vi "Aux CO2 Serial Check.vi"(11 "?":T1={"Serial Port"={"termination char"=10, "End read on termination character?"=TRUE, "Enabled?"=FALSE, "VISA resource name"="COM1", "baud rate"=9600, "data bits"=8, "parity"=enum."None", "stop bits"=10, "flow control"=0, "timeout (ms)"=10000, "Input buffer size"=4096, "End write on termination character?"=TRUE, "XON Char"=17, "XOFF Char"=19}, "Baro Pressure"=760, "Device"=0} {"Device" items=["None", "TidalWave", "LoFlow / Canary", "Capnogard"]; "Serial Port"."XOFF Char" format="%.0x"; "Serial Port"."XON Char" format="%.0x"; "Serial Port"."flow control" items=["None"=0, "XON/XOFF"=1, "RTS/CTS"=2, "DTR/DSR"=4]; "Serial Port"."stop bits" items=["1.0"=10, "1.5"=15, "2.0"=20]; "Serial Port"."data bits" min=5 max=8 step=1; "Serial Port"."baud rate" items=["75"=75, "110"=110, "134"=134, "150"=150, "300"=300, "600"=600, "1200"=1200, "1800"=1800, "2400"=2400, "4800"=4800, "7200"=7200, "9600"=9600, "14400"=14400, "19200"=19200, "28800"=28800, "38400"=38400, "56000"=56000, "57600"=57600, "115200"=115200, "128000"=128000, "230400"=230400]; "Serial Port"."termination char" format="%.0x"}) -> ()   [LabVIEW 2016]
uses:
  Controls/Aux CO2 Diags.ctl
  Controls/Aux CO2 Selector.ctl
  Controls/Aux CO2 Control.ctl
  Controls/Serial Visa Control.ctl
  Controls/SerialPortControl.ctl
  Miscellaneous/Globals.vi
panel:
  in  "Set Comps":bool
  in  "Settings Cmd":bool
  in  "Zero Cmd":bool
  in  "Poff Cmd":bool
  in  "Pon Cmd":bool
  in  "Start Cmd":bool
  in  "Stop Cmd":bool
  in  "Stop Button":bool
  out "Serial Data (Hex)":string
  out "Serial Data (ASCII)":string
  out "Waveform Chart":sgl(graph)
  out "Ready to Log 2":bool
  out "Ref. Capnometer Port":T4={"Port"="", "Source"=0, "Active"=FALSE, "Baro Pressure"=760, "SerialRxBuffer"="", "Raw CO2 (Torr)"=5.0, "bytes read"=5, "Status"=[], "Status Message"=enum.""} {"Status" format="%x"; "Raw CO2 (Torr)" format="%.2f"; "Baro Pressure" min=400 max=800; "Source" items=["None", "TidalWave", "LoFlow / Canary", "Capnogard"]}
  out "Init OK":bool
  # "LoFlo Specific Commands"
  # "mmHg"
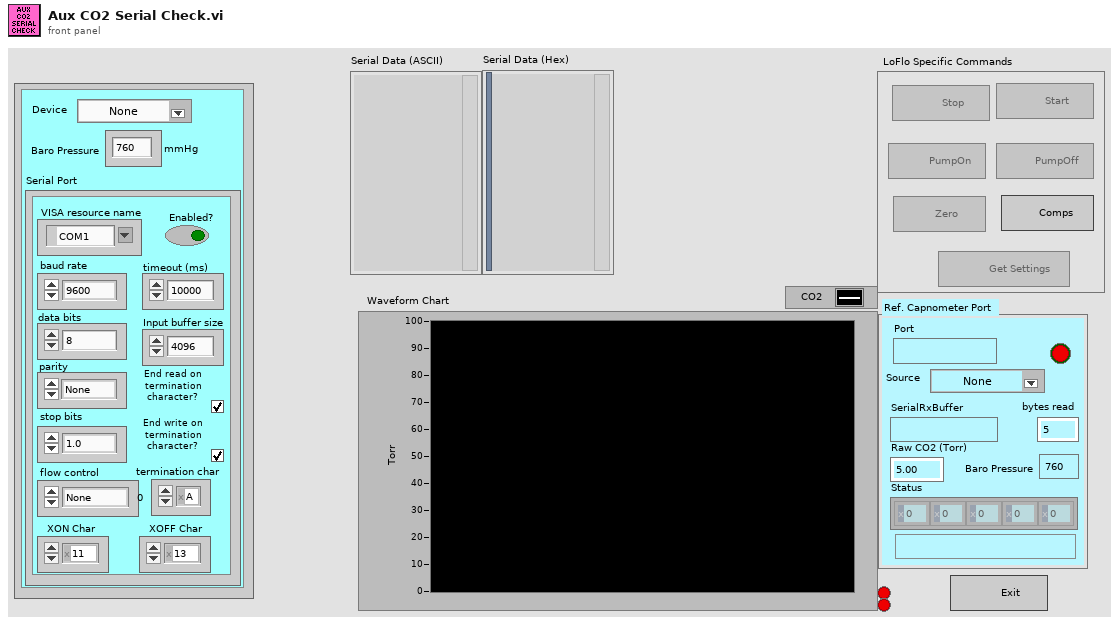
[diagram p1: front panel]
types:
  T1 = typedef "Aux CO2 Control.ctl" = cluster{"Serial Port":T2, "Baro Pressure":u32, "Device":T3}
  T2 = typedef "Serial Visa Control.ctl" = cluster{"termination char":u8, "End read on termination character?":bool, "Enabled?":bool, "VISA resource name":refnum<visa-resource-name>, "baud rate":u32, "data bits":u16, "parity":enum16{"None", "Odd", "Even", "Mark", "Space"}, "stop bits":u16, "flow control":u16, "timeout (ms)":u32, "Input buffer size":u32, "End write on termination character?":bool, "XON Char":u8, "XOFF Char":u8}
  T3 = typedef "Aux CO2 Selector.ctl" = u16
  T4 = typedef "Aux CO2 Diags.ctl" = cluster{"Port":refnum<visa-resource-name>, "Source":T3, "Active":bool, "Baro Pressure":u16, "SerialRxBuffer":string, "Raw CO2 (Torr)":sgl, "bytes read":i16, "Status":u8[], "Status Message":enum16{"", "Sensor Over Temp", "Sensor Faulty", "Set BaroP", "Capno in Sleep Mode", "Zero In Progress", "Sensor Warm Up", "Check Sampling Line", "Zero Required", "CO2 Out Of Range", "Check Airway Adapter", "LoFlo Not Connected"}}
  T5 = enum8{"Enabled", "Disabled", "Disabled and Grayed Out"}
  T6 = typedef "SerialPortControl.ctl" = enum16{"Initialize", "Write Data", "Read Data", "Close Port"}
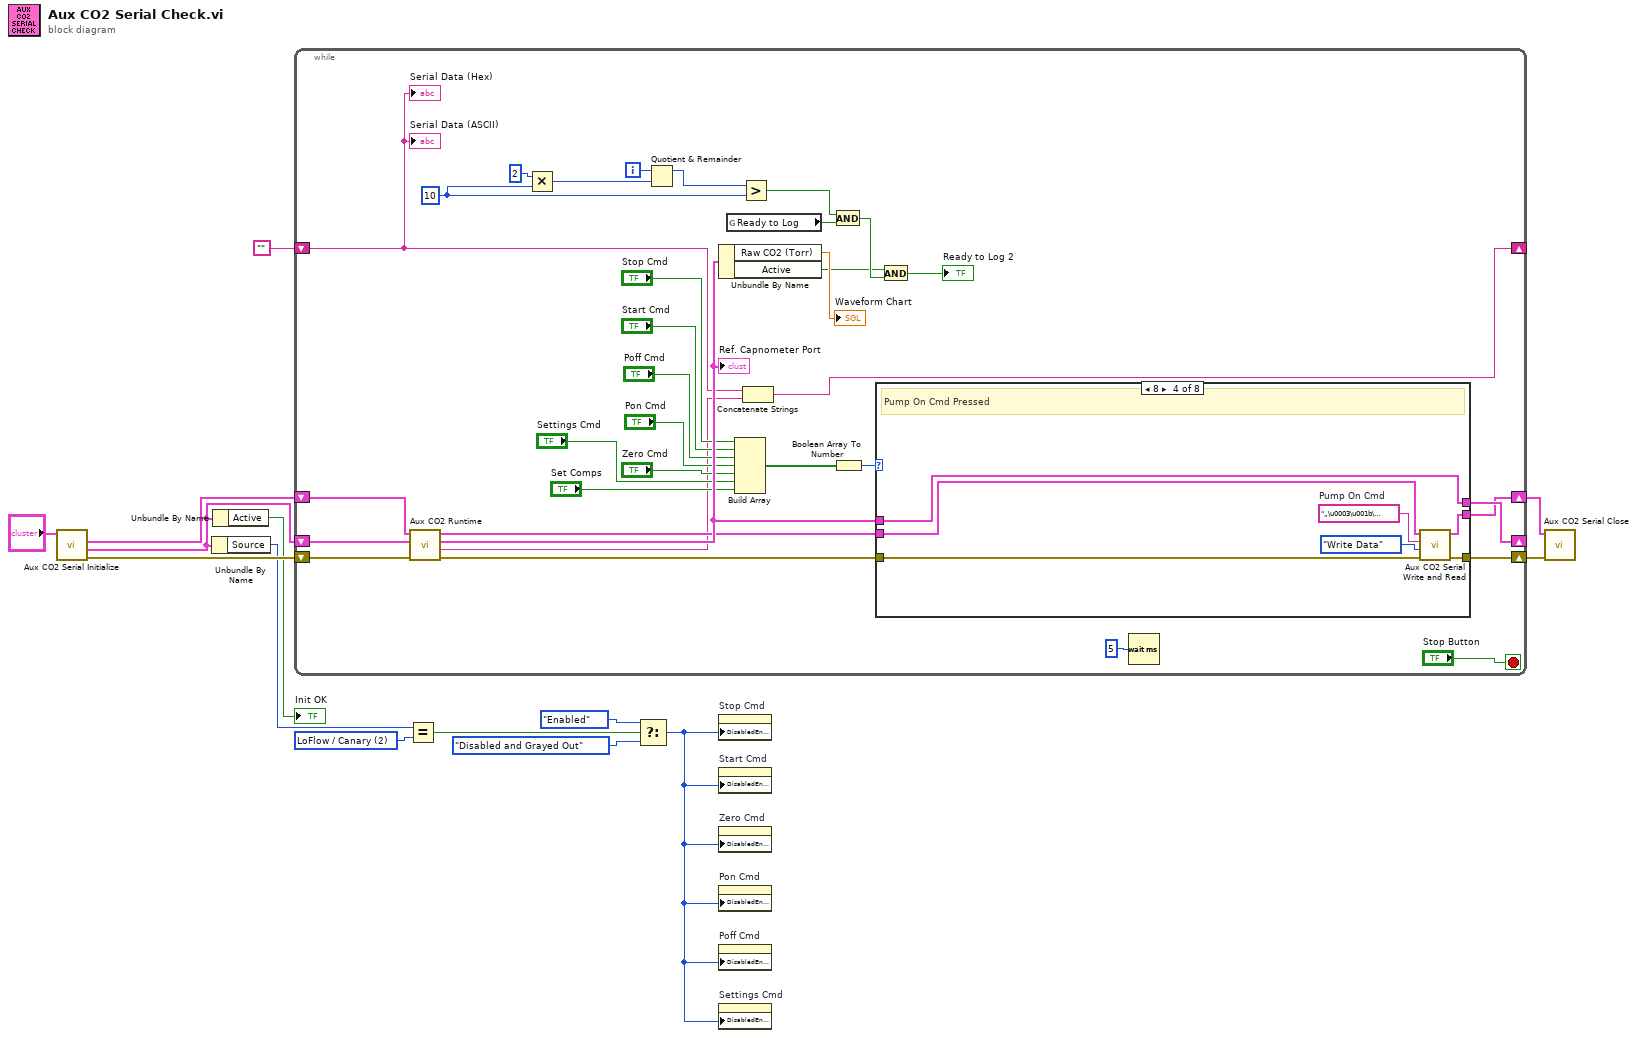
[diagram p0: block diagram]
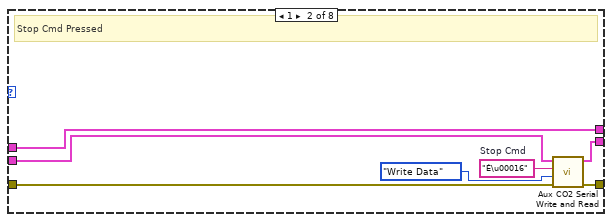
[diagram p3: hidden frame]
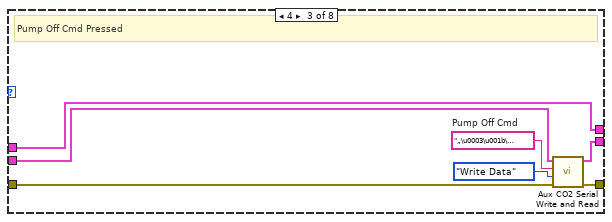
[diagram p4: hidden frame]
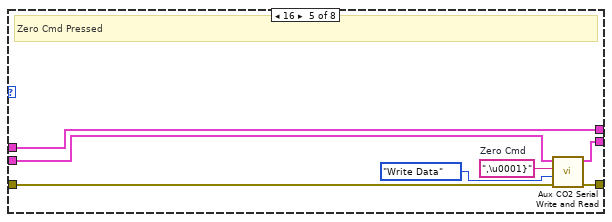
[diagram p5: hidden frame]
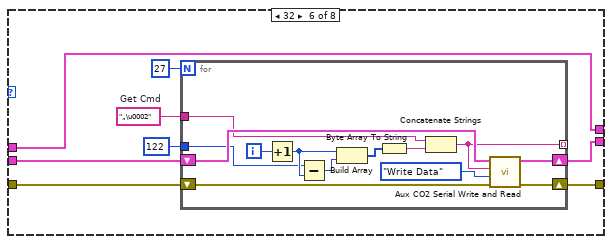
[diagram p6: hidden frame]
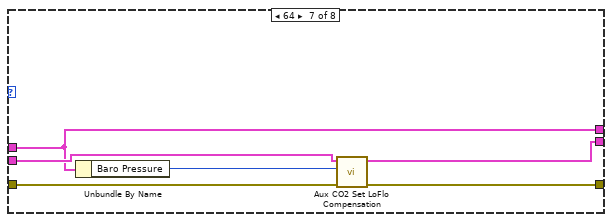
[diagram p7: hidden frame]
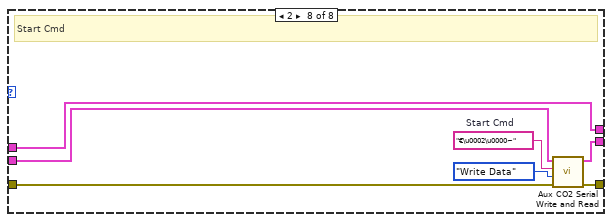
[diagram p8: hidden frame]
diagram:
  w8 = T3 2 items=["None", "TidalWave", "LoFlow / Canary", "Capnogard"] ("y")
  n1 = call "Aux CO2 Serial Initialize.vi"("CO2 Channel"="?") -> ("error Out"=w14:errorcluster, "output cluster"=w4:T4, "Serial Port Out"=w13:T2)  [unwired: 8 in]
  n2 = Unbundle By Name(w4) -> ("Source"=w9:T3)
  n3 = Unbundle By Name(w4) -> ("Active"=→"Init OK":bool)
  n4 = while {
    shift-right: [w34] -> _
    shift-left: w4 -> [w39]
    shift-right: [w32] -> w10
    shift-left: w13 -> [w41]
    shift-right: [w36] -> w11
    shift-left: w14 -> [w40]
    shift-right: [w37] -> _
    shift-left: "" -> [w19]
    i -> [w46]
    stop <- "Stop Button" stop-if-true
    w45 = 10
    n5 = call "Aux CO2 Runtime.vi"("Error In"=w40, "Capno Data In"=w39, "Serial Port In"=w41) -> ("Error Out"=w35:errorcluster, "RawBytesRead"=w20:string, "Capno Data Out"=w33:T4, "Serial Port Out"=w31:T2)  [unwired: 5 in]
    "Ref. Capnometer Port" <- w33
    n6 = Multiply(x=2, y=w45) -> (x*y=w44:i32)
    n7 = Quotient & Remainder(x=w46, y=w44) -> (x-y*floor(x/y)=w47:i32)  [unwired: 1 out]
    n8 = Unbundle By Name(w33) -> ("Raw CO2 (Torr)"=→"Waveform Chart":sgl, "Active"=w17:bool)
    n9 = global read "Globals.vi" "Ready to Log"() -> (w15:bool)
    n10 = Build Array("Stop Cmd", "Start Cmd", "Poff Cmd", "Pon Cmd", "Zero Cmd", "Settings Cmd", "Set Comps") -> (w29:bool[])
    n11 = Greater?(x=w47, y=w45) -> (0:w42:bool)
    n12 = Concatenate Strings(w19, w20) -> (w37:string)
    n13 = And(x=w42, y=w15) -> (x .and. y?=w18:bool)
    n14 = Boolean Array To Number(Boolean array=w29) -> (number=w26:u32)
    n15 = case shown="8" w26 {
      tunnel: w35 -> [w51 w54 w61 w68 w75 w87 w104 w110]
      tunnel: [w51 w53 w60 w67 w74 w84 w103 w109] -> w36
      tunnel: w33 -> [w50 w58 w65 w72 w79 w83 w102 w107]
      tunnel: [w50 w58 w65 w72 w79 w83 w102 w107] -> w34
      tunnel: w31 -> [w49 w55 w62 w69 w76 w86 w106 w111]
      tunnel: [w49 w52 w59 w66 w73 w85 w105 w108] -> w32
      frame 0, Default {
        # "No Button Pressed"
      }
      frame 1 {
        w57 = "É\u00016"  # Stop Cmd
        # "Stop Cmd Pressed"
        n16 = call "Aux CO2 Serial Write and Read.vi"("error in"=w54, "Action"=SerialPortControl."Write Data", "string to write"=w57, "Serial Port"=w55) -> ("error IO"=w53:errorcluster, "Serial Port Out"=w52:T2)  [unwired: 2 out]
      }
      frame 4 {
        w64 = "„\u0003\u001b\u0001]"  # Pump Off Cmd
        # "Pump Off Cmd Pressed"
        n17 = call "Aux CO2 Serial Write and Read.vi"("error in"=w61, "Action"=SerialPortControl."Write Data", "string to write"=w64, "Serial Port"=w62) -> ("error IO"=w60:errorcluster, "Serial Port Out"=w59:T2)  [unwired: 2 out]
      }
      frame 8 {
        w71 = "„\u0003\u001b\u0000^"  # Pump On Cmd
        # "Pump On Cmd Pressed"
        n18 = call "Aux CO2 Serial Write and Read.vi"("error in"=w68, "Action"=SerialPortControl."Write Data", "string to write"=w71, "Serial Port"=w69) -> ("error IO"=w67:errorcluster, "Serial Port Out"=w66:T2)  [unwired: 2 out]
      }
      frame 16 {
        w78 = "‚\u0001}"  # Zero Cmd
        # "Zero Cmd Pressed"
        n19 = call "Aux CO2 Serial Write and Read.vi"("error in"=w75, "Action"=SerialPortControl."Write Data", "string to write"=w78, "Serial Port"=w76) -> ("error IO"=w74:errorcluster, "Serial Port Out"=w73:T2)  [unwired: 2 out]
      }
      frame 32 {
        w81 = "„\u0002"  # Get Cmd
        n20 = for {
          N: 27 -> [_]
          shift-right: [w97] -> w85
          shift-left: w86 -> [w98]
          shift-right: [w96] -> w84
          shift-left: w87 -> [w99]
          tunnel: w81 -> [w95]
          tunnel: u8 122 -> [w89]
          tunnel: [w88] -> _ mode=indexing
          i -> [w94]
          n21 = Increment(x=w94) -> (x+1=w90:i32)
          n22 = Subtract(x=w89, y=w90) -> (x-y=w91:i32)
          n23 = Build Array(w90, w91) -> (w93:i32[])
          n24 = Byte Array To String(unsigned byte array=w93) -> (string=w92:string)
          n25 = Concatenate Strings(w95, w92) -> (w88:string)
          n26 = call "Aux CO2 Serial Write and Read.vi"("error in"=w99, "Action"=SerialPortControl."Write Data", "string to write"=w88, "Serial Port"=w98) -> ("error IO"=w96:errorcluster, "Serial Port Out"=w97:T2)  [unwired: 2 out]
        }
      }
      frame 64 {
        n27 = Unbundle By Name(w102) -> ("Baro Pressure"=w101:u16)
        n28 = call "Aux CO2 Set LoFlo Compensation.vi"("error In"=w104, "Baro Pressure"=w101, "Serial Port In"=w106) -> ("error Out"=w103:errorcluster, "Serial Port Out"=w105:T2)  [unwired: 7 in]
      }
      frame 2 {
        w112 = "€\u0002\u0000~"  # Start Cmd
        # "Start Cmd"
        n29 = call "Aux CO2 Serial Write and Read.vi"("error in"=w110, "Action"=SerialPortControl."Write Data", "string to write"=w112, "Serial Port"=w111) -> ("error IO"=w109:errorcluster, "Serial Port Out"=w108:T2)  [unwired: 2 out]
      }
    }
    n30 = And(x=w17, y=w18) -> (x .and. y?=→"Ready to Log 2":bool)
    n31 = Wait (ms)(milliseconds to wait=u32 5) -> ()  [unwired: 1 out]
    "Serial Data (Hex)" <- w19
    "Serial Data (ASCII)" <- w19
  }
  n32 = Equal?(x=w9, y=w8) -> (x = y?=w7:bool)
  n33 = Select(t=T5."Enabled" ("Disabled"), s=w7, f=T5."Disabled and Grayed Out" ("Disabled")) -> (s? t:f=w1:T5)
  n34 = property on="Stop Cmd" class="Bool"("DisabledEnum"=w1) -> ()  [unwired: 2 in, 2 out]
  n35 = property on="Start Cmd" class="Bool"("DisabledEnum"=w1) -> ()  [unwired: 2 in, 2 out]
  n36 = property on="Zero Cmd" class="Bool"("DisabledEnum"=w1) -> ()  [unwired: 2 in, 2 out]
  n37 = property on="Pon Cmd" class="Bool"("DisabledEnum"=w1) -> ()  [unwired: 2 in, 2 out]
  n38 = property on="Poff Cmd" class="Bool"("DisabledEnum"=w1) -> ()  [unwired: 2 in, 2 out]
  n39 = property on="Settings Cmd" class="Bool"("DisabledEnum"=w1) -> ()  [unwired: 2 in, 2 out]
  n40 = call "Aux CO2 Serial Close.vi"("error in"=w11, "Serial Port In"=w10) -> ()  [unwired: 7 in, 3 out]
